vi "Data Type for Instrument.vi"(1 "Inst type":T2=enum."Raw with zero offsetting") -> (0 "Data for Inst Type":T1)   [LabVIEW 2022 SP3]
uses:
  Controls/Inst_type.ctl
  Controls/Data for Inst Type.ctl
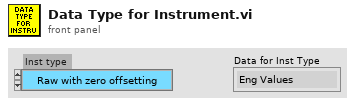
[diagram p1: front panel]
types:
  T1 = typedef "Data for Inst Type.ctl" = enum16{"Eng Values", "Voltage"}
  T2 = typedef "Inst_type.ctl" = enum16{"Raw voltage", "Raw with zero offsetting", "Propeller anemometer", "Pressure Transducer", "Pitot-static tube", "Hot wire", "Cross wire 1", "Cross wire 2", "Generic Linear", "Generic Polynomial", "Generic BackPoly", "Fast FID", "Thermocouple", "Cold wire", "Pulsed Wire", "LDA Vel", "LDA Tran time", "LDA Arr time", "Microphone"}
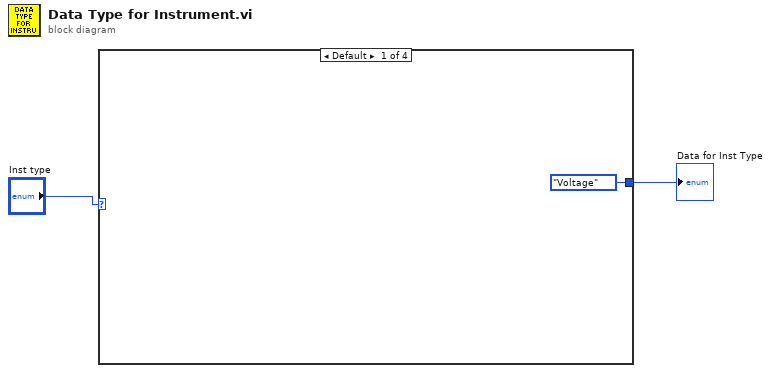
[diagram p0: block diagram]
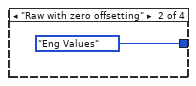
[diagram p2: hidden frame]
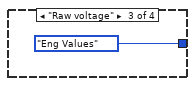
[diagram p3: hidden frame]
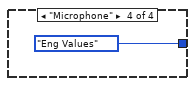
[diagram p4: hidden frame]
diagram:
  n1 = case shown="Default" "Inst type" {
    tunnel: [Data_for_Inst_Type."Voltage" ("Data for Inst Type") Data_for_Inst_Type."Eng Values" ("Data for Inst Type") Data_for_Inst_Type."Eng Values" ("Data for Inst Type") Data_for_Inst_Type."Eng Values" ("Data for Inst Type")] -> w1
    frame Default {
    }
    frame "Raw with zero offsetting" {
    }
    frame "Raw voltage" {
    }
    frame "Microphone" {
    }
  }
  "Data for Inst Type" <- w1
